vi "Send_String.vi"(8 "error in (no error)":errorcluster, 10 "String":string, 11 "SpinCoater in":refnum<class "SpinCoater.lvclass">) -> (0 "error out":errorcluster, 2 "read buffer":string, 3 "SpinCoater out":refnum<class "SpinCoater.lvclass">)   [LabVIEW 2020, in "SpinCoater.lvclass"]
uses:
  <instrlib>/Classes/SpinCoater/SpinCoater.lvclass
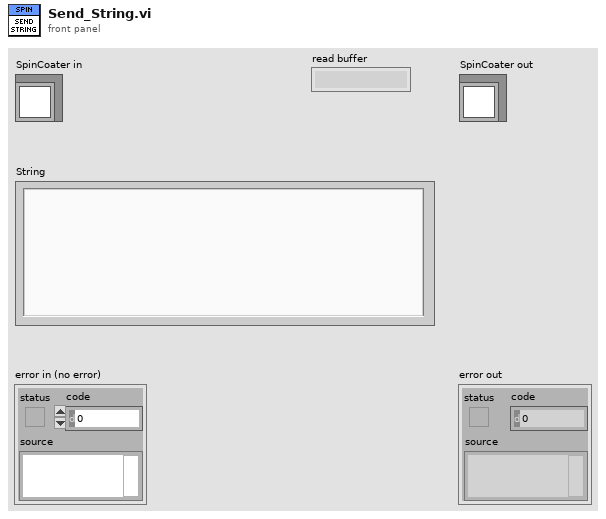
[diagram p1: front panel]
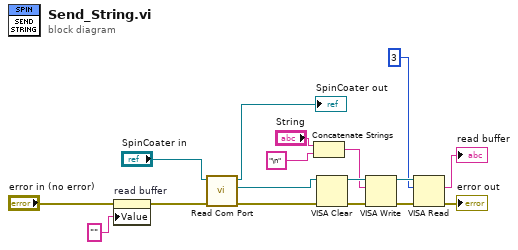
[diagram p0: block diagram]
diagram:
  n1 = property on="read buffer" class="Str"(error in="error in (no error)", "Value"="" ("read buffer")) -> (error out=w4:errorcluster)  [unwired: 1 in, 1 out]
  n2 = call-dynamic "Read Com Port.vi"("error in (no error)"=w4, "SpinCoater in"="SpinCoater in") -> ("error out"=w12:errorcluster, "Com Port"=w15:refnum<visa-resource-name>, "SpinCoater out"=→"SpinCoater out":refnum<class "SpinCoater.lvclass">)  [unwired: 7 in]
  n3 = Concatenate Strings("String", "\n") -> (w1:string)
  n4 = VISA Clear(VISA resource name=w15, error in (no error)=w12) -> (VISA resource name out=w14:refnum<visa-resource-name>, error out=w13:errorcluster)
  n5 = VISA Write(VISA resource name=w14, write buffer=w1, error in (no error)=w13) -> (VISA resource name out=w11:refnum<visa-resource-name>, error out=w10:errorcluster)  [unwired: 1 out]
  n6 = VISA Read(VISA resource name=w11, byte count=u32 3, error in (no error)=w10) -> (read buffer=→"read buffer":string, error out=→"error out":errorcluster)  [unwired: 2 out]
